vi "Configure Channel.vi"(4 "Bandwidth (0: MAX Bandwidth)":i32(ring) items=["MAX Bandwidth", "Unlimited"], 5 "Channel (0: Channel 1)":i32(ring) items=["Channel 1", "Channel 2", "Channel 3", "Channel 4", "Math", "Reference A", "Reference B", "Reference C", "Reference D"], 6 "Vertical Offset (0.0 divs)":dbl, 7 "Vertical Coupling (1: DC)":i32(ring)=1 items=["AC", "DC", "Ground"], 8 "error in (no error)":errorcluster, 9 "Vertical Range (10.0 V/div)":dbl=10.0, 10 "Probe Attenuation (10: 10X)":i32(ring)=10 items=["1"=1, "10"=10, "20"=20, "50"=50, "100"=100, "500"=500, "1000"=1000], 11 "Osciloscope in":refnum<class "Osciloscope.lvclass">) -> (0 "error out":errorcluster, 3 "Osciloscope out":refnum<class "Osciloscope.lvclass">)   [LabVIEW 2020, in "Osciloscope Tektronix.lvlib" / "Osciloscope.lvclass"]
uses:
  Osciloscope.lvclass
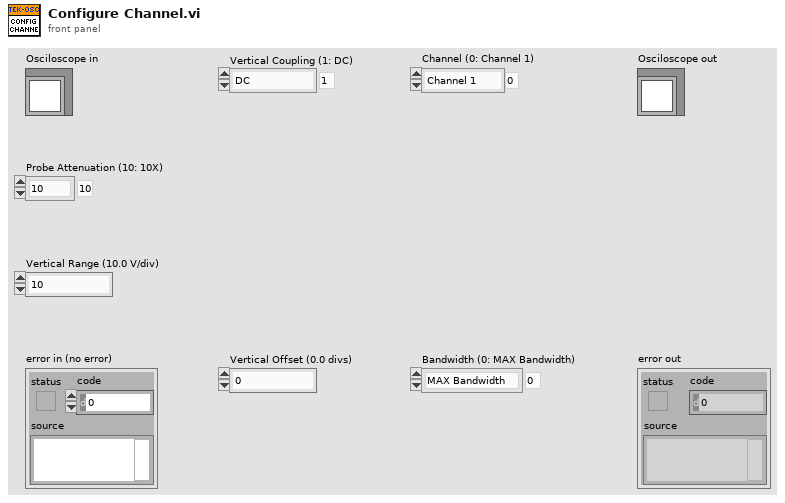
[diagram p1: front panel]
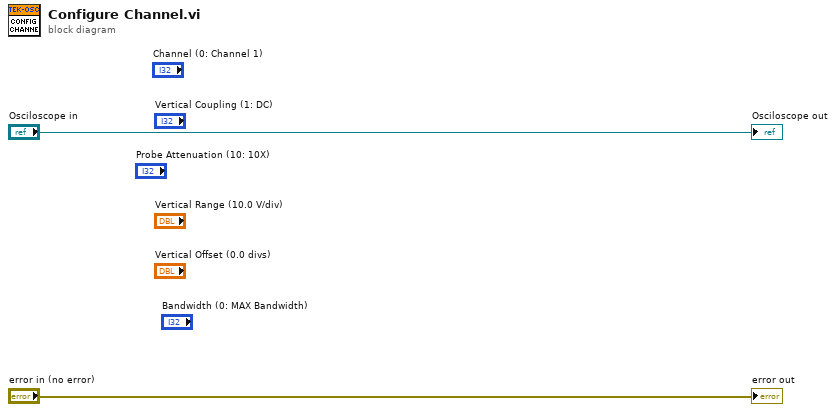
[diagram p0: block diagram]
diagram:
  "error out" <- "error in (no error)"
  "Osciloscope out" <- "Osciloscope in"
